vi "test-Encrypt (FFT - mismatch Multiplier).vi"(8 "error in (no error)":errorcluster, 11 "TestCase in":refnum<class "Test-Encryption.lvclass">=refnum) -> (0 "error out":errorcluster, 3 "TestCase out":refnum<class "Test-Encryption.lvclass">)   [LabVIEW 2019, in "Test-Encryption.lvclass"]
uses:
  Test-Encryption.lvclass
  Encryption/Encryption.lvclass
  Encryption/FFT/FFT.lvclass
  Layouts/Layout.lvclass
  C:/Development/Open Source/tsc-event-logger/Encryption/Encryption.lvclass
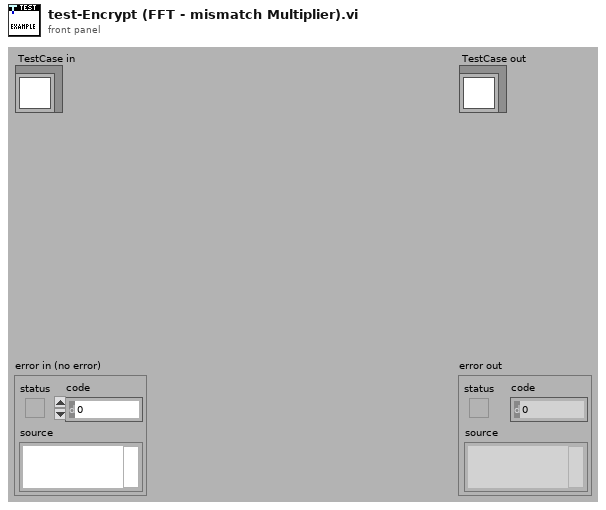
[diagram p1: front panel]
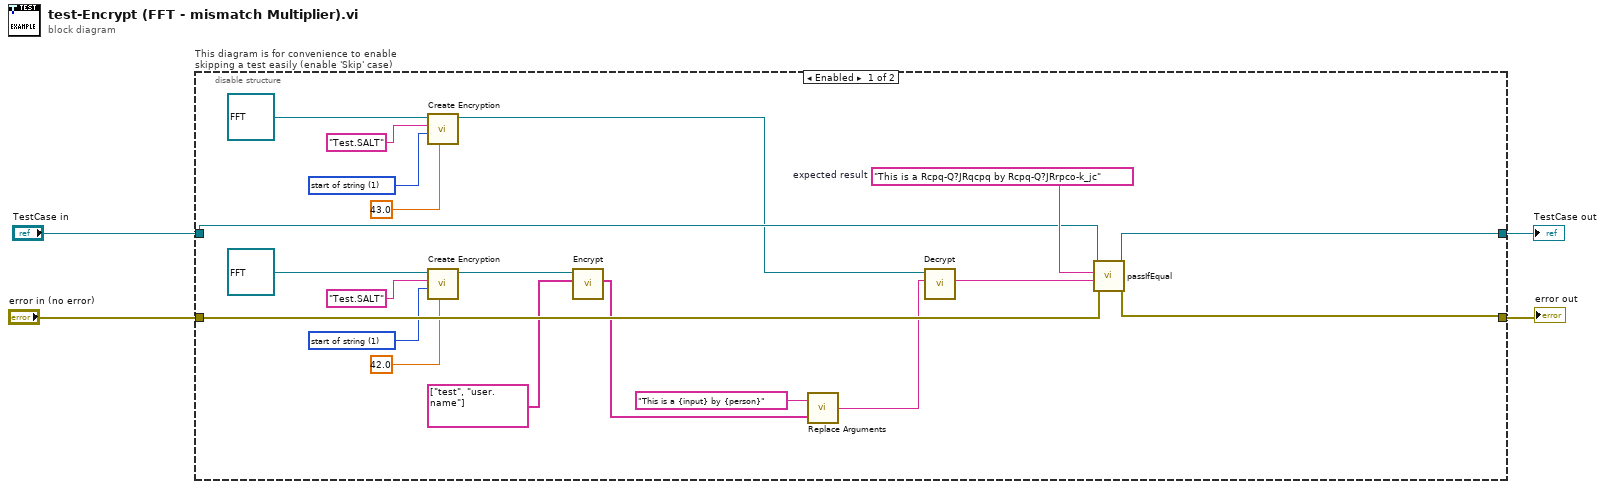
[diagram p0: block diagram]
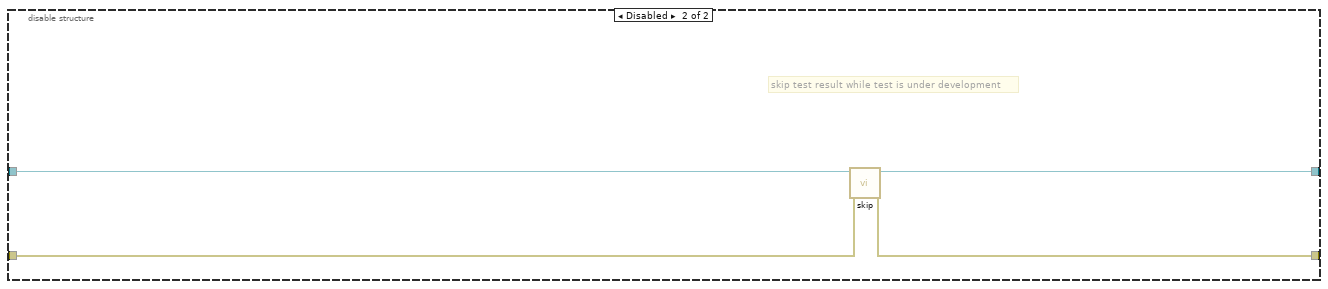
[diagram p2: hidden frame]
diagram:
  n1 = disable-structure "This diagram is for convenience to enable skipping a test easily (enable 'Skip' case)" shown="Enabled" {
    disable-tunnel: "TestCase in" -> [w23 w28]
    disable-tunnel: [w22 w26] -> w1
    disable-tunnel: [w21 w27] -> w3
    disable-tunnel: "error in (no error)" -> [w20 w25]
    frame Enabled {
      w8 = u16 1 items=["both", "start of string", "end of string"] ("SALT location (start of string)")
      w17 = u16 1 items=["both", "start of string", "end of string"] ("SALT location (start of string)")
      w24 = "This is a Rcpq-Q?JRqcpq by Rcpq-Q?JRrpco-k_jc"  # expected result
      n2 = call "Create Encryption.vi"("Multiplier"=43.0, "SALT location (start of string)"=w8, "SALT"="Test.SALT", "Encryption Method"=refnum<class "FFT.lvclass"> refnum ("TSC Event Logger.lvlib:FFT.lvclass")) -> ("Encryption output"=w5:refnum<class "FFT.lvclass">)  [unwired: 6 in, 1 out]
      n3 = call "Create Encryption.vi"("Multiplier"=42.0, "SALT location (start of string)"=w17, "SALT"="Test.SALT", "Encryption Method"=refnum<class "FFT.lvclass"> refnum ("TSC Event Logger.lvlib:FFT.lvclass")) -> ("Encryption output"=w15:refnum<class "FFT.lvclass">)  [unwired: 6 in, 1 out]
      n4 = call-dynamic "Encrypt.vi"("Arguments"=string[] ["test", "user.name"], "FFT in"=w15) -> ("Encrypted Arguments"=w12:string[])  [unwired: 7 in, 2 out]
      n5 = call "Replace Arguments.vi"("Arguments"=w12, "Message"="This is a {input} by {person}") -> ("Output Message"=w11:string)
      n6 = call-dynamic "Decrypt.vi"("Message"=w11, "FFT in"=w5) -> ("Decrypted Message"=w10:string)  [unwired: 7 in, 2 out]
      n7 = call-dynamic "passIfEqual.vi"("error in (no error)"=w20, "y"=w10, "x"=w24, "TestCase in"=w23) -> ("error out"=w21:errorcluster, "TestCase out"=w22:refnum<class "Test-Encryption.lvclass">)  [unwired: 6 in]
    }
    frame Disabled {
      # "skip test result while test is under development"
      n8 = call <vilib>:"skip.vi"("error in (no error)"=w25, "TestCase in"=w28) -> ("error out"=w27:errorcluster, "TestCase out"=w26:refnum<class "Test-Encryption.lvclass">)  [unwired: 8 in]
    }
  }
  "error out" <- w3
  "TestCase out" <- w1
